vi "RichToFlatpumploop_GetValveRequest.vi"(5 "OutputClusterType":T1, 11 "InputCluster":T2) -> (3 "OutputCluster":T1)   [LabVIEW 2024, in "pumploop_client.lvlib"]
uses:
  pumploop_client.lvlib
  pumploop_GetValveRequest.ctl
  pumploop_GetValveRequest_Flat.ctl
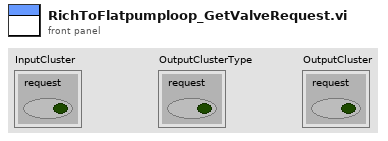
[diagram p1: front panel]
types:
  T1 = typedef "pumploop_client.lvlib/pumploop_GetValveRequest_Flat.ctl" = cluster{"request":bool}
  T2 = typedef "pumploop_client.lvlib/pumploop_GetValveRequest.ctl" = cluster{"request":bool}
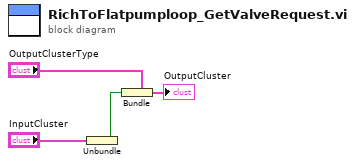
[diagram p0: block diagram]
diagram:
  n1 = Unbundle "Unbundle"("InputCluster") -> ("request"=w1:bool)
  n2 = Bundle "Bundle"(cluster="OutputClusterType", "request"=w1) -> (→"OutputCluster":T1)
